vi "File.Split 1D array to N row 2D array.vi"(9 "Divider":i32, 11 "Files":path[](array[path])) -> (3 "Files Out":path[][](array[path]))   [LabVIEW 2018]
panel:
  out "size(s)":i32[](array[numeric])
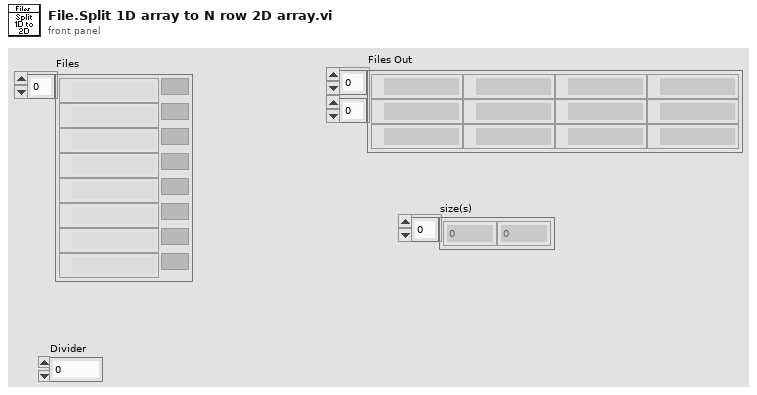
[diagram p1: front panel]
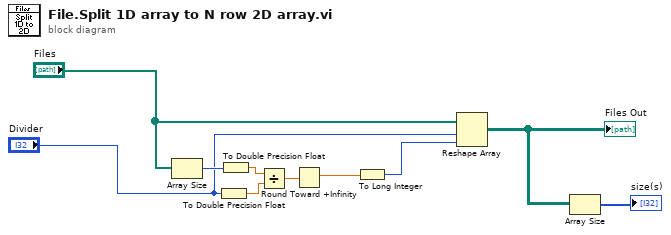
[diagram p0: block diagram]
diagram:
  n1 = Array Size(array="Files") -> (size(s)=w7:i32)
  n2 = To Double Precision Float(number="Divider") -> (double precision float=w5:dbl)
  n3 = To Double Precision Float(number=w7) -> (double precision float=w6:dbl)
  n4 = Divide(x=w6, y=w5) -> (x/y=w4:dbl)
  n5 = Round Toward +Infinity(x=w4) -> (ceil(x): smallest int >= x=w3:dbl)
  n6 = To Long Integer(number=w3) -> (32bit integer=w2:i32)
  n7 = Reshape Array("Files", "Divider", w2) -> (w10:path[][])
  "Files Out" <- w10
  n8 = Array Size(array=w10) -> (size(s)=→"size(s)":i32[])
